vi "Metrolab Digital Integrator.vi"(1 "Action":T3=enum."Identify", 2 "Parameters":variant) -> (6 "Output":variant, 7 "Stop":bool)   [LabVIEW 2019]
uses:
  Sub Controls/Instrument Actions.ctl
  Sub Controls/Public.ctl
  Sub Controls/Instrument Match.ctl
  Sub Controls/Scan Output.ctl
  Sub Controls/Instrument IDN.ctl
  Sub Controls/User Event Command.ctl
panel:
  in  "Gain":i16(slide)=1 min=0 max=9 step=1 scale=0.0..9.0
  out "Old Reading":dbl
  out "# Overflows":dbl
  in  "Reset":bool
  out "Title":string="Metrolab Digital Integrator"
  in  "VISA resource name":refnum<visa-resource-name>
  in  "Instruments":T1[](array[typedef])=[{"Model"="PDI5025", "Manufacturer"="METROLAB SA Geneva", "Term Character"="", "Wait Time (mS)"=0, "Wait for SRQ"=FALSE, "Type"="Digital Integrator"}]
  out "Model":string
  in  "Address":u16(ring)
  in  "Public":T2
  out "Measurement":dbl[](array[numeric]) format="%^.3e"
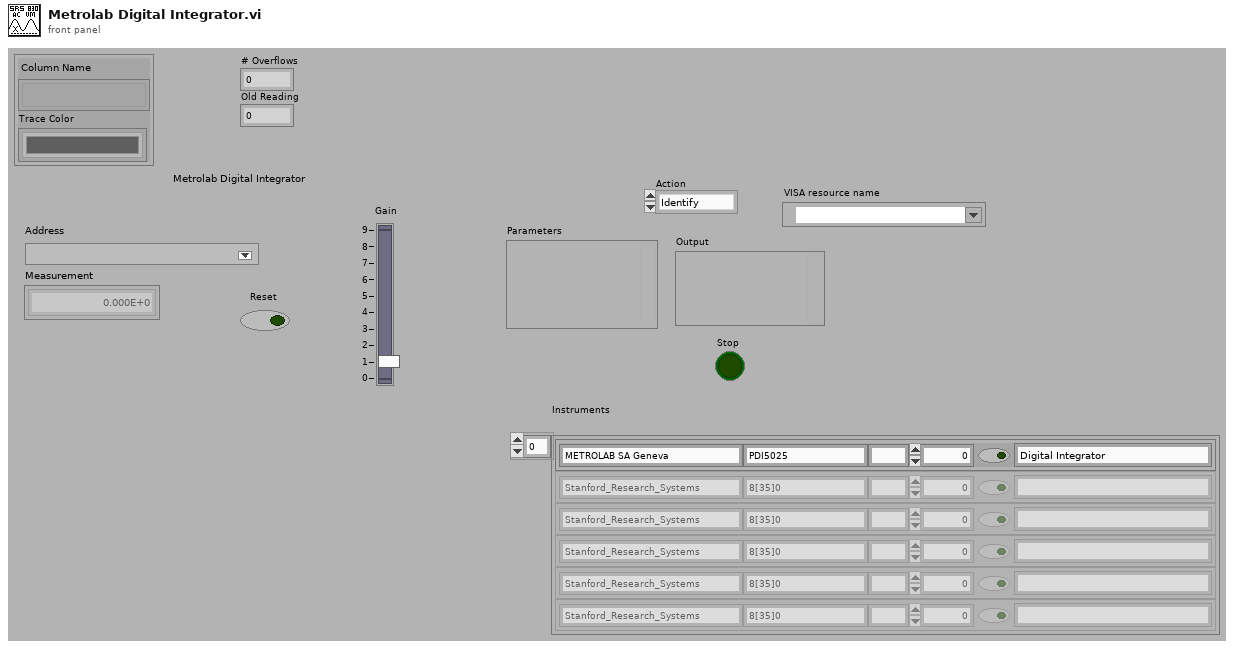
[diagram p1: front panel]
types:
  T1 = typedef "Instrument Match.ctl" = cluster{"Model":string, "Manufacturer":string, "Term Character":string, "Wait Time (mS)":u32, "Wait for SRQ":bool, "Type":string}
  T2 = typedef "Public.ctl" = cluster{"Column Name":string[], "Trace Color":u32[]}
  T3 = typedef "Instrument Actions.ctl" = enum16{"Scan", "Identify", "New", "Configure", "Initialize", "Test", "Read", "Close"}
  T4 = typedef "Scan Output.ctl" = cluster{"Manufacturer":string, "Model":string, "Info":string, "Revision":string, "error out":errorcluster}
  T5 = typedef "Instrument IDN.ctl" = cluster{"VISA Address":string, "Status":u16, "Manufacturer":string, "Model":string, "Info":string, "Info 2":string, "Misc Data":variant}
  T6 = typedef "User Event Command.ctl" = enum32{"Stop Config"}
  T7 = cluster{"VISA resource name":refnum<visa-resource-name>, string}
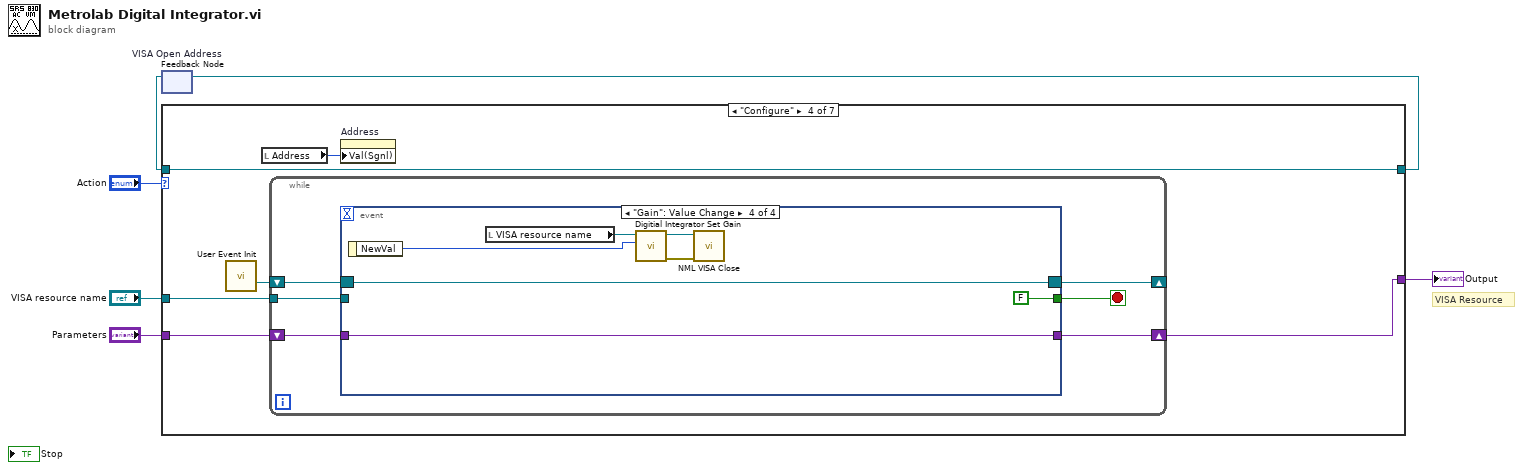
[diagram p0: block diagram]
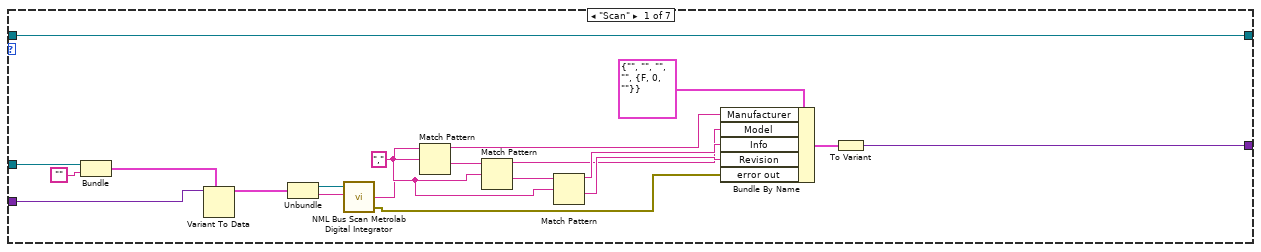
[diagram p2: hidden frame]
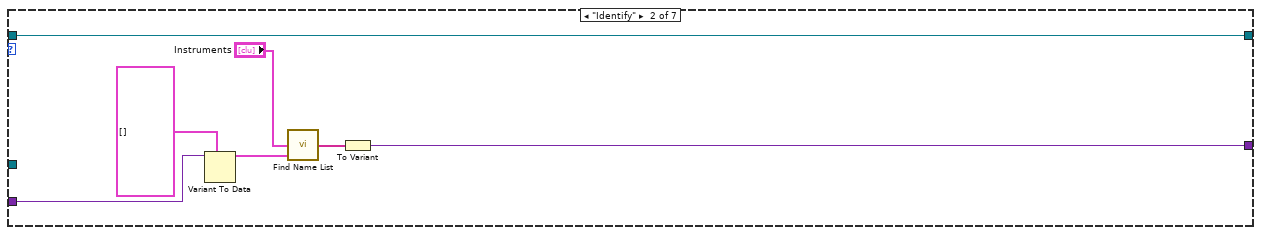
[diagram p3: hidden frame]
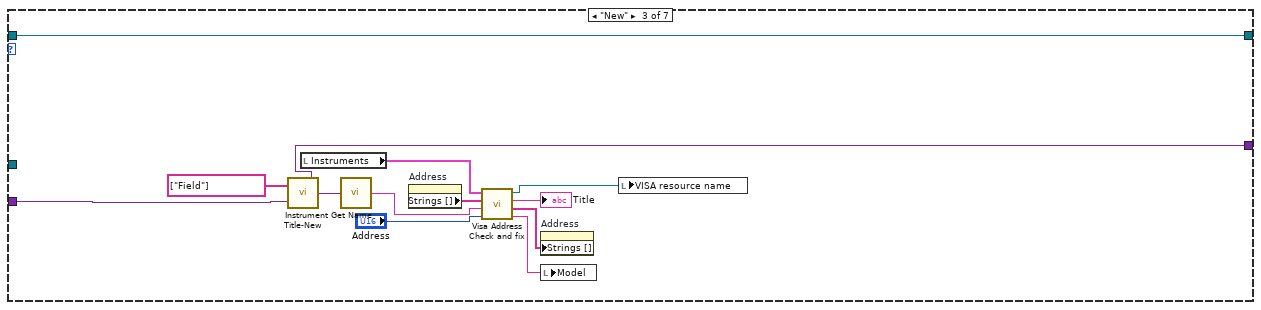
[diagram p4: hidden frame]
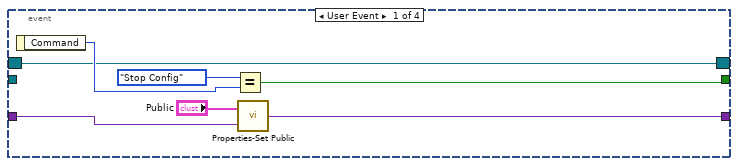
[diagram p5: hidden frame]
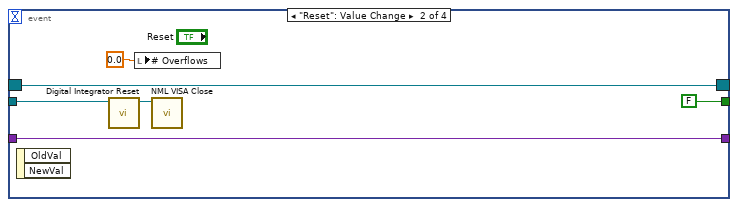
[diagram p6: hidden frame]
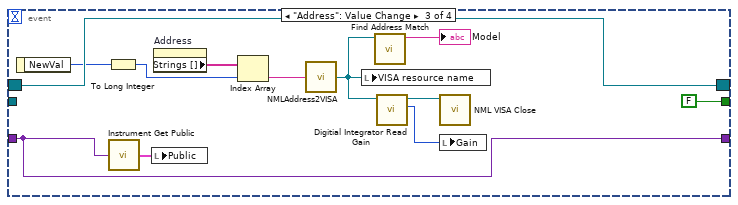
[diagram p7: hidden frame]
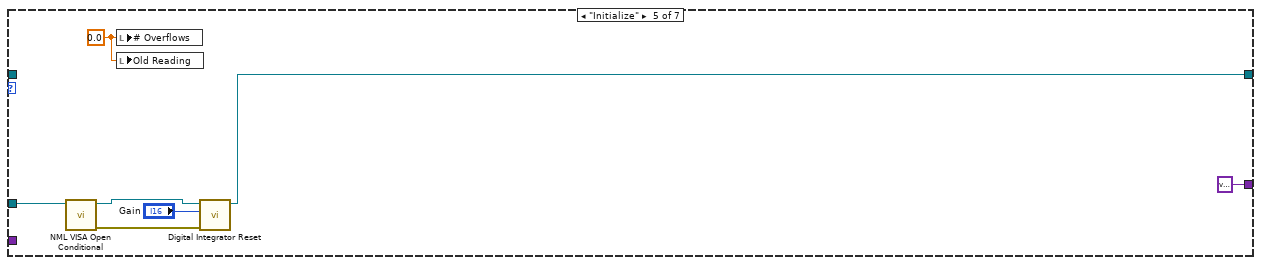
[diagram p8: hidden frame]
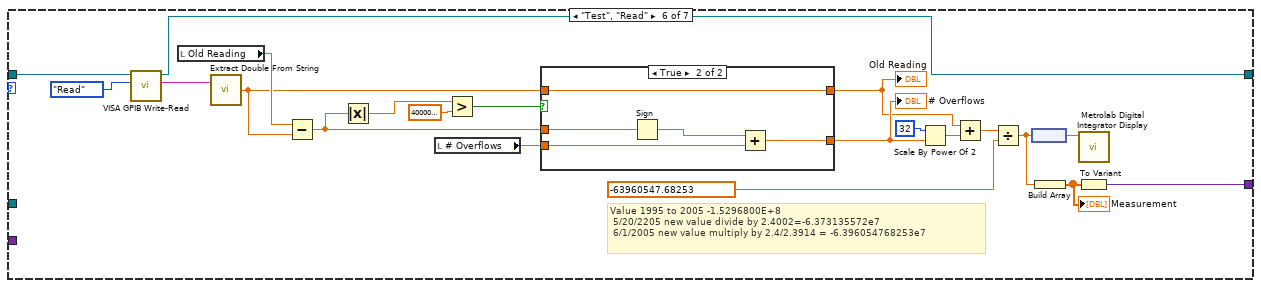
[diagram p9: hidden frame]
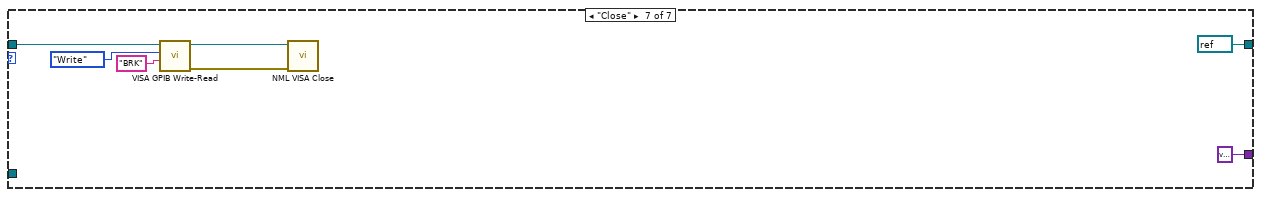
[diagram p11: hidden frame]
diagram:
  # "VISA Resource"
  n1 = feedback #1 "VISA Open Address"() -> (w3:refnum<visa-resource-name>)  [unwired: 1 in]
  n2 = case shown="\"Configure\"" "Action" {
    tunnel: [w26 w33 w34 w47 w94 w109 refnum<visa-resource-name> refnum ("Open VISA Resource name")] -> w4
    tunnel: w3 -> [w26 w33 w34 w47 _ w110 w125]
    tunnel: [w25 w32 w37 w49 variant ("Variant") w117 variant ("Variant")] -> w6
    tunnel: "VISA resource name" -> [w24 _ _ w46 w90 _ _]
    tunnel: "Parameters" -> [w7 w27 w35 w48 _ _ _]
    frame "Scan" {
      w18 = ","
      n3 = Bundle("VISA resource name"=w24, "") -> (w22:T7)  [unwired: 1 in]
      n4 = Variant To Data(type=w22, Variant=w7) -> (data=w21:T7)  [unwired: 1 in, 1 out]
      n5 = Unbundle(w21) -> ("VISA resource name"=w11:refnum<visa-resource-name>, w10:string)
      n6 = call "NML Bus Scan Metrolab Digital Integrator.vi"("String Read In"=w10, "VISA Session"=w11) -> ("error out"=w8:errorcluster, "String Read Out"=w9:string)  [unwired: 1 in, 1 out]
      n7 = Match Pattern(string=w9, regular expression=w18) -> (before substring=w13:string, after substring=w20:string)  [unwired: 1 in, 2 out]
      n8 = Match Pattern(string=w20, regular expression=w18) -> (before substring=w14:string, after substring=w19:string)  [unwired: 1 in, 2 out]
      n9 = Match Pattern(string=w19, regular expression=w18) -> (before substring=w15:string, after substring=w16:string)  [unwired: 1 in, 2 out]
      n10 = Bundle By Name(cluster=T4 {"Manufacturer"="", "Model"="", "Info"="", "Revision"="", "error out"={"status"=FALSE, "code"=0, "source"=""}} ("Scan Output"), "Manufacturer"=w13, "Model"=w14, "Info"=w15, "Revision"=w16, "error out"=w8) -> (w12:T4)
      n11 = To Variant(anything=w12) -> (Variant=w25:variant)
    }
    frame "Identify" {
      n12 = Variant To Data(type=T5[] [], Variant=w27) -> (data=w29:T5[])  [unwired: 1 in, 1 out]
      n13 = call "Find Name List.vi"("Bus Scan"=w29, "Instruments"="Instruments") -> ("Names"=w28:string[])  [unwired: 1 in]
      n14 = To Variant(anything=w28) -> (Variant=w32:variant)
    }
    frame "New" {
      n15 = call "Title-New.vi"("Parameters"=w35, "Array"=string[] ["Field"]) -> ("Instrument Prop"=w37:variant)
      n16 = local read "Instruments"() -> (w39:T1[])
      n17 = call "Instrument Get Name.vi"("Parameters"=w37) -> ("Type"=w41:string)
      n18 = property on="Address" class="Ring (strict)"() -> ("Strings []"=w43:string[])  [unwired: 2 in, 2 out]
      n19 = call "Visa Address Check and fix.vi"("Address"="Address", "Name"=w41, "NML Addresses"=w43, "Instruments"=w39) -> ("Model"=w38:string, "NML Addresses"=w42:string[], "Title"=→"Title":string, "VISA resource name"=w36:refnum<visa-resource-name>)  [unwired: 2 out]
      n20 = property on="Address" class="Ring (strict)"("Strings []"=w42) -> ()  [unwired: 2 in, 2 out]
      n21 = local write "Model"(w38) -> ()
      n22 = local write "VISA resource name"(w36) -> ()
    }
    frame "Configure" {
      n23 = call "User Event Init.vi"() -> ("Event Registration Refnum"=w51:refnum<event-registration>)  [unwired: 14 in, 1 out]
      n24 = local read "Address"() -> (w50:u16)
      n25 = while {
        shift-right: [w57] -> w49
        shift-left: w48 -> [w56]
        shift-right: [w53] -> _
        shift-left: w51 -> [w54]
        tunnel: w46 -> [w52]
        stop <- w55 stop-if-true
        n26 = event shown="[3] \"Gain\": Value Change" {
          selector: w54 -> [w58 w66 w82 w88]
          dyn-events: [w58 w66 w82 w88] -> w53
          timeout: _ -> [_ _ _ _]
          tunnel: [w60 FALSE FALSE FALSE] -> w55
          tunnel: w56 -> [w63 w67 w72 w89]
          tunnel: [w64 w67 w72 w89] -> w57
          tunnel: w52 -> [_ w70 _ _]
          event User Event {
            n27 = event-data() -> ("Command"=w62:T6)  [unwired: 1 in]
            n28 = Equal?(x=User_Event_Command."Stop Config", y=w62) -> (x = y?=w60:bool)
            n29 = call "Properties-Set Public.vi"("Variant"=w63, "New Public"="Public") -> ("Variant 2"=w64:variant)
          }
          event "Reset": Value Change {
            n30 = event-data() -> ()  [unwired: 1 in, 2 out]
            n31 = call "Digital Integrator Reset.vi"("VISA resource name"=w70) -> ("VISA resource name"=w69:refnum<visa-resource-name>)  [unwired: 10 in]
            n32 = local write "# Overflows"(0.0 ("# Overflows")) -> ()
            n33 = call "NML VISA Close.vi"("VISA resource name"=w69) -> ()  [unwired: 10 in, 1 out]
          }
          event "Address": Value Change {
            n34 = event-data() -> ("NewVal"=w80:u16)  [unwired: 1 in]
            n35 = To Long Integer(number=w80) -> (32bit integer=w76:i32)
            n36 = call "Instrument Get Public.vi"("Variant"=w72) -> ("Public"=w71:T2)
            n37 = local write "Public"(w71) -> ()
            n38 = property on="Address" class="Ring (strict)"() -> ("Strings []"=w79:string[])  [unwired: 2 in, 2 out]
            n39 = Index Array(array=w79, index=w76) -> (element=w78:string)
            n40 = call "NMLAddress2VISA.vi"("NML Address"=w78) -> ("VISA resource name"=w75:refnum<visa-resource-name>)
            n41 = local write "VISA resource name"(w75) -> ()
            n42 = call "Find Address Match.vi"("VISA resource name"=w75) -> ("Model"=→"Model":string)  [unwired: 3 in, 3 out]
            n43 = call "Digitial Integrator Read Gain.vi"("VISA resource name"=w75) -> ("Gain"=w73:i16, "VISA resource name dup"=w74:refnum<visa-resource-name>)  [unwired: 8 in, 1 out]
            n44 = call "NML VISA Close.vi"("VISA resource name"=w74) -> ()  [unwired: 10 in, 1 out]
            n45 = local write "Gain"(w73) -> ()
          }
          event "Gain": Value Change {
            n46 = event-data() -> ("NewVal"=w85:i16)  [unwired: 1 in]
            n47 = local read "VISA resource name"() -> (w86:refnum<visa-resource-name>)
            n48 = call "Digitial Integrator Set Gain.vi"("Gain"=w85, "VISA resource name"=w86) -> ("error out"=w83:errorcluster, "VISA resource name dup"=w84:refnum<visa-resource-name>)  [unwired: 8 in]
            n49 = call "NML VISA Close.vi"("Error In"=w83, "VISA resource name"=w84) -> ()  [unwired: 9 in, 1 out]
          }
        }
      }
      n50 = property on="Address" class="Ring (strict)"("Val(Sgnl)"=w50) -> ()  [unwired: 2 in, 2 out]
    }
    frame "Initialize" {
      w93 = 0.0 ("# Overflows")
      n51 = call "NML VISA Open Conditional.vi"("VISA resource name"=w90) -> ("error out"=w92:errorcluster, "dup VISA Session"=w95:refnum<visa-resource-name>)  [unwired: 8 in, 1 out]
      n52 = local write "# Overflows"(w93) -> ()
      n53 = local write "Old Reading"(w93) -> ()
      n54 = call "Digital Integrator Reset.vi"("error in (no error)"=w92, "Gain"="Gain", "VISA resource name"=w95) -> ("VISA resource name"=w94:refnum<visa-resource-name>)  [unwired: 8 in]
    }
    frame "Test", "Read" {
      # "Value 1995 to 2005 -1.5296800E+8\n 5/20/2205 new value divide by 2.4002=-6.373135572e7\n 6/1/2005 new value multiply by 2.4/2.3914 = -6.396054768253e7"
      n55 = call "VISA GPIB Write-Read.vi"("Action"=enum16{"Write", "Read", "Write & Read"}."Read", "VISA resource name"=w110) -> ("String Returned"=w111:string, "dup VISA Session"=w109:refnum<visa-resource-name>)  [unwired: 6 in, 2 out]
      n56 = local read "Old Reading"() -> (w106:dbl)
      n57 = call "Extract Double From String.vi"("string"=w111) -> ("floating pt. number"=w101:dbl)  [unwired: 1 in, 2 out]
      n58 = Subtract(x=w106, y=w101) -> (x-y=w102:dbl)
      n59 = Absolute Value(x=w102) -> (abs(x)=w105:dbl)
      n60 = local read "# Overflows"() -> (w107:dbl)
      n61 = Greater?(x=w105, y=4000000000.0) -> (0:w103:bool)
      n62 = case shown="True" w103 {
        tunnel: w102 -> [_ w124]
        tunnel: w107 -> [w119 w122]
        tunnel: [w119 w121] -> w115
        tunnel: w101 -> [w118 w120]
        tunnel: [w118 w120] -> w100
        frame False {
        }
        frame True {
          n63 = Sign(1:w124) -> (0:w123:dbl)
          n64 = Add(x=w123, y=w122) -> (x+y=w121:dbl)
        }
      }
      "# Overflows" <- w115
      "Old Reading" <- w100
      n65 = Scale By Power Of 2(n=32, x=w115) -> (x*2^n=w113:dbl)
      n66 = Add(x=w100, y=w113) -> (x+y=w112:dbl)
      n67 = Divide(x=w112, y=-63960547.68253) -> (x/y=w98:dbl)
      n68 = node(w98) -> (w97:dbl[unit])
      n69 = Build Array(w98) -> (w99:dbl[])
      "Measurement" <- w99
      n70 = call "Metrolab Digital Integrator Display.vi"("Field"=w97) -> ()  [unwired: 11 in]
      n71 = To Variant(anything=w99) -> (Variant=w117:variant)
    }
    frame "Close" {
      n72 = call "VISA GPIB Write-Read.vi"("Command"="BRK", "Action"=enum16{"Write", "Read", "Write & Read"}."Write", "VISA resource name"=w125) -> ("error out"=w126:errorcluster, "dup VISA Session"=w127:refnum<visa-resource-name>)  [unwired: 5 in, 2 out]
      n73 = call "NML VISA Close.vi"("Error In"=w126, "VISA resource name"=w127) -> ()  [unwired: 9 in, 1 out]
    }
  }
  "Output" <- w6
  n74 = feedback-in #1(w4) -> ()
